vi "main.vi"() -> ()   [LabVIEW 2020]
uses:
  Var/Queue elements.ctl
  Var/Queue elements 2.ctl
  Var/Global 1.vi
  user32.dll
panel:
  out "Примерное время \nобработки":string
  out "2_stan":refnum<queue>
  out "Flag":bool
  out "Curs":refnum<queue>
  out "Progress":i32(slide) scale=-1.0..500.0
  in  "Количество брака":i32 caption="Numeric"
  in  "Общее кол-во обработок":i32 caption="Numeric"
  in  "Close":bool
  out "ERROR":string
  out "Boolean":bool
  in  "Start":bool
  in  "Stop":bool
  in  "error in (no error)":errorcluster
  out "error out":errorcluster
  in  "Объекты":T1={"Ускоренно/Реально"=TRUE, "Станок 1"={"Время на обработку (с)"=40, "Шанс брака (%)"=4.0}, "Станок 2"={"Время на обработку (с)"=60, "Шанс брака (%)"=8.0}, "Кол-во деталей"=500, "Задержки на перемещение"={"Время загрузки\n первого станка (с)"=5, "Время загрузки\n второго станка (с) "=6, "Время до урны (с)"=3, "Время до коробки (с)"=2, "Время между станками (с)"=3}, "Повторная \nобработка\n на станке:"=TRUE}
  # "1"
  # "2"
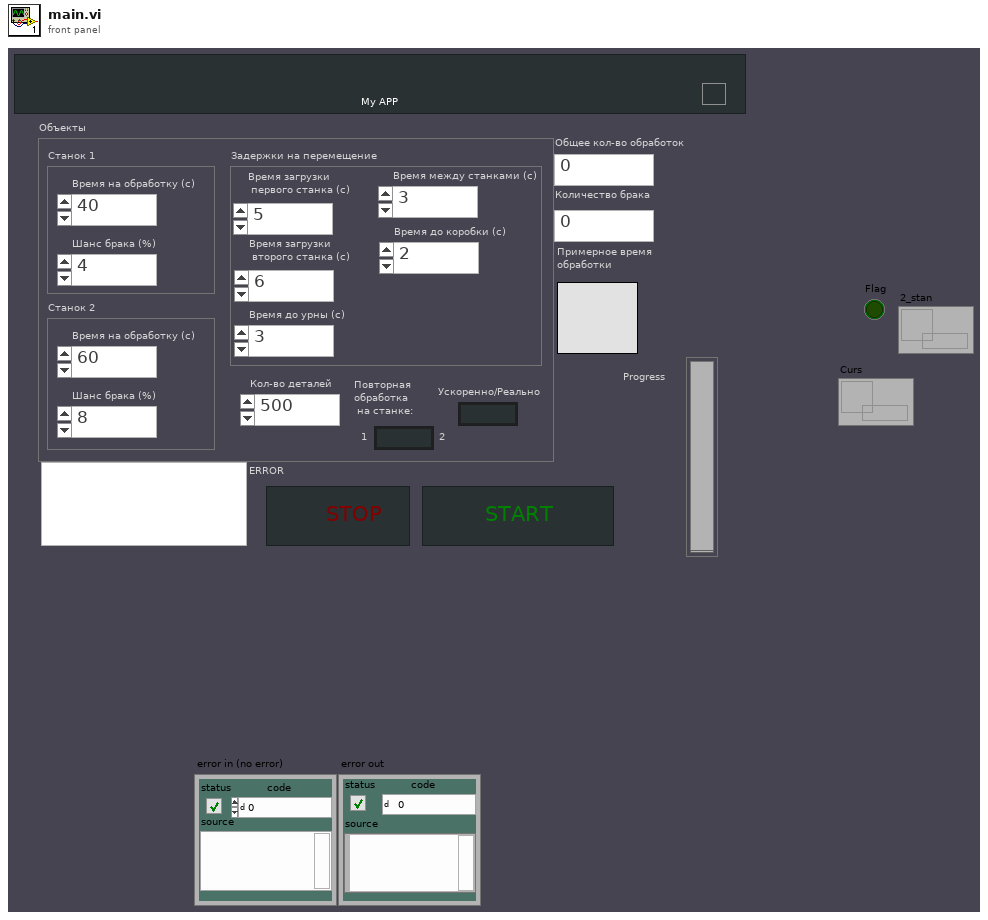
[diagram p1: front panel]
types:
  T1 = cluster{"Ускоренно/Реально":bool, "Станок 1":cluster{"Время на обработку (с)":i32, "Шанс брака (%)":dbl}, "Станок 2":cluster{"Время на обработку (с)":i32, "Шанс брака (%)":dbl}, "Кол-во деталей":i32, "Задержки на перемещение":cluster{"Время загрузки\n первого станка (с)":i32, "Время загрузки\n второго станка (с) ":i32, "Время до урны (с)":i32, "Время до коробки (с)":i32, "Время между станками (с)":i32}, "Повторная \nобработка\n на станке:":bool}
  T2 = typedef "Queue elements 2.ctl" = enum16{"START", "STOP", "CLOSE", "CLEAR"}
  T3 = typedef "Queue elements.ctl" = enum16{"STOP", "START", "CLOSE"}
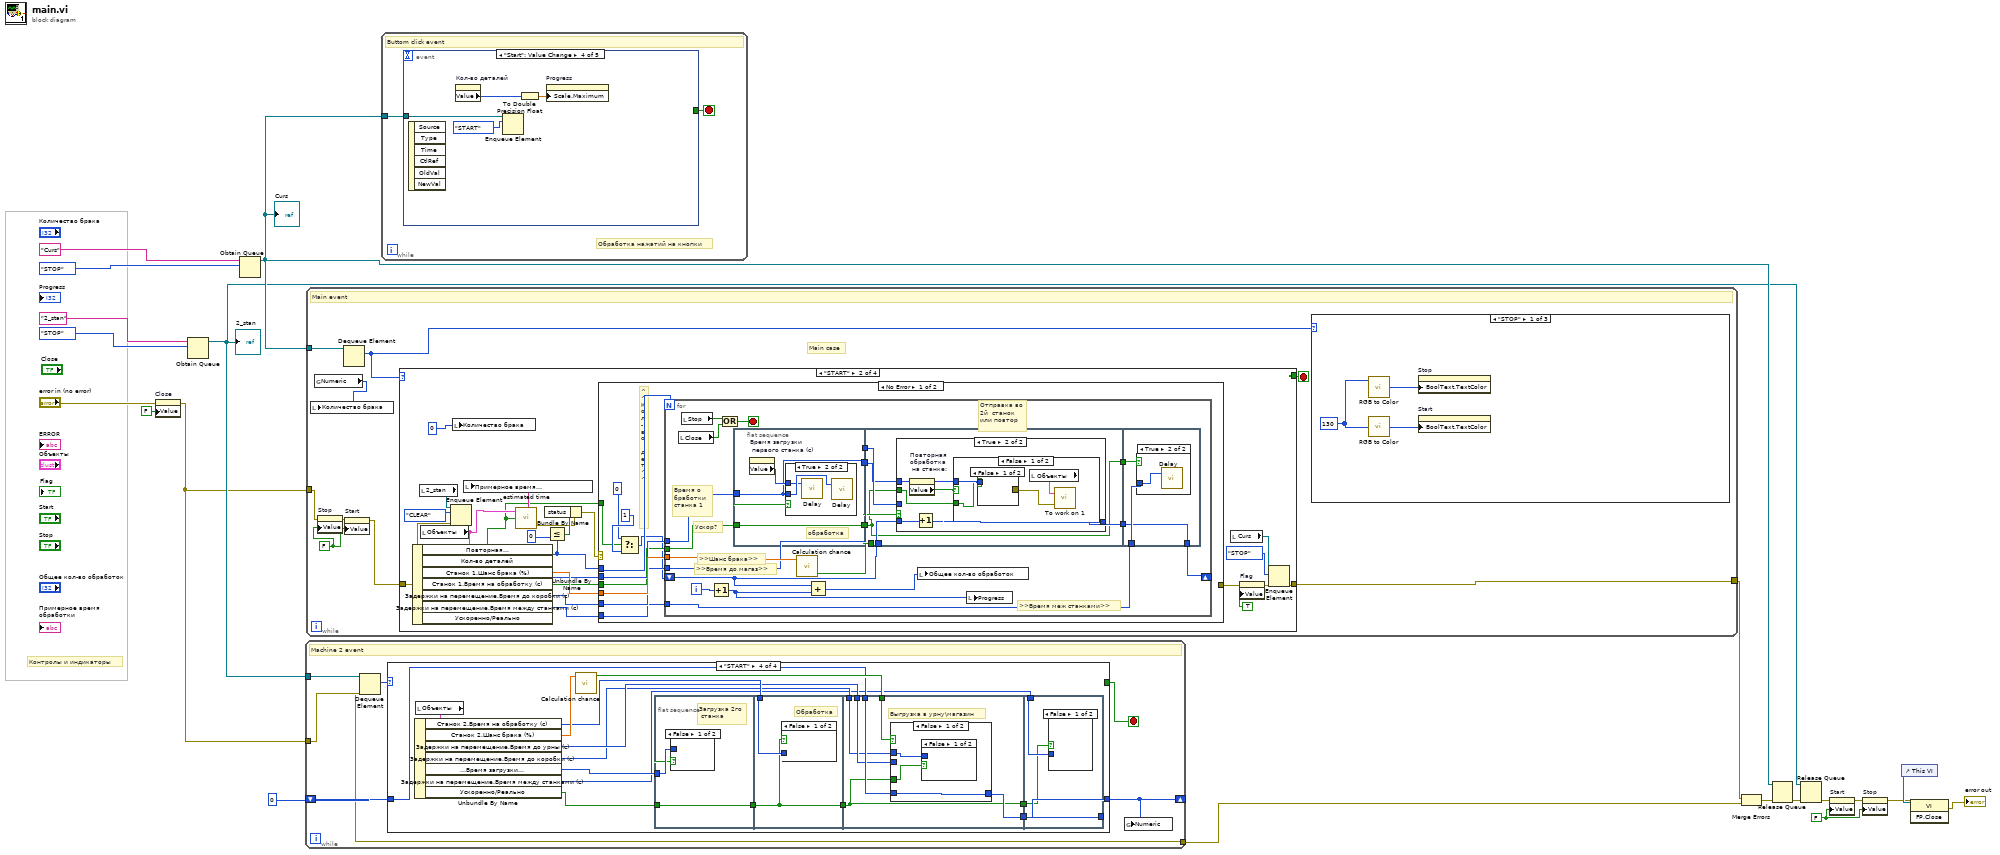
[diagram p0: block diagram]
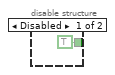
[diagram p3: hidden frame]
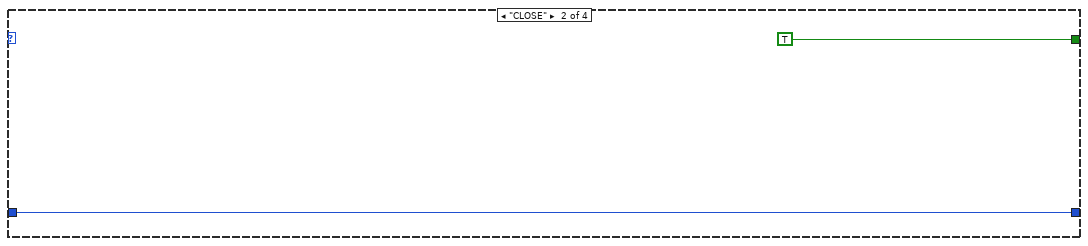
[diagram p4: hidden frame]
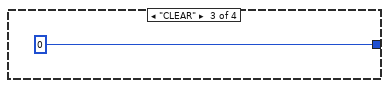
[diagram p5: hidden frame]
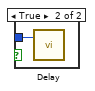
[diagram p6: hidden frame]
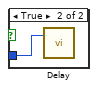
[diagram p7: hidden frame]
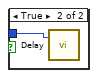
[diagram p8: hidden frame]
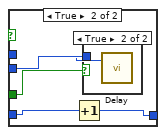
[diagram p9: hidden frame]
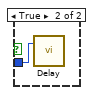
[diagram p11: hidden frame]
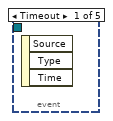
[diagram p12: hidden frame]
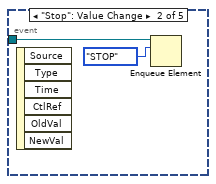
[diagram p13: hidden frame]
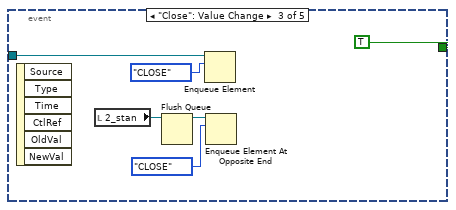
[diagram p14: hidden frame]
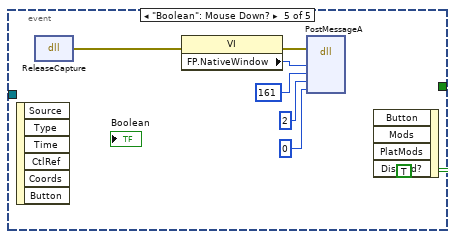
[diagram p15: hidden frame]
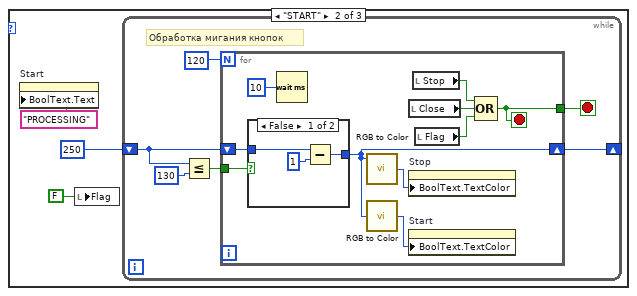
[diagram p16: hidden frame]
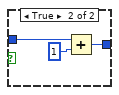
[diagram p17: hidden frame]
diagram:
  w16 = FALSE ("Text Only Button")
  # "Контролы и индикаторы"
  n1 = property on="Close" class="Bool (strict)"(error in="error in (no error)", "Value"=FALSE ("Close")) -> (error out=w5:errorcluster)  [unwired: 1 in, 1 out]
  n2 = Obtain Queue(name (unnamed)="2_stan", element data type=Queue_elements_2."STOP" ("element")) -> (queue out=w9:refnum<queue>)  [unwired: 3 in, 2 out]
  "2_stan" <- w9
  n3 = Obtain Queue(name (unnamed)="Curs", element data type=Queue_elements."STOP") -> (queue out=w18:refnum<queue>)  [unwired: 3 in, 2 out]
  "Curs" <- w18
  n4 = while {
    tunnel: w9 -> [w25]
    shift-right: [w21] -> _
    shift-left: 0 -> [w24]
    tunnel: [w22] -> w6
    tunnel: w5 -> [w23]
    stop <- w26 stop-if-true
    # "Machine 2 event"
    n5 = Dequeue Element(queue=w25, error in (no error)=w23) -> (element=w27:T2, error out=w22:errorcluster)  [unwired: 1 in, 2 out]
    n6 = case shown="\"START\"" w27 {
      tunnel: [w29 TRUE _ _] -> w26
      tunnel: w24 -> [w28 w31 _ w44]
      tunnel: [w28 w31 0 w41] -> w21
      frame "STOP" {
        n7 = disable-structure shown="Enabled" {
          disable-tunnel: [TRUE _] -> w29
          frame Disabled {
          }
          frame Enabled {
          }
        }
      }
      frame "CLOSE" {
      }
      frame "CLEAR" {
      }
      frame "START" {
        n8 = local read "Объекты"() -> (w48:T1)
        n9 = Unbundle By Name(w48) -> ("Станок 2.Время на обработку (с)"=w46:i32, "Станок 2.Шанс брака (%)"=w47:dbl, "Задержки на перемещение.Время до урны (с)"=w43:i32, "Задержки на перемещение.Время до коробки (с)"=w42:i32, "Задержки на перемещение.Время загрузки\n второго станка (с)"=w40:i32, "Задержки на перемещение.Время между станками (с)"=w38:i32, "Ускоренно/Реально"=w34:bool)
        n10 = call "Calculation chance.vi"("Defective (%)"=w47) -> ("Defect"=w45:bool)  [unwired: 1 in]
        n11 = flat-sequence {
          tunnel: w40 -> [w50]
          tunnel: w34 -> [w49]
          tunnel: [w49] -> w37
          tunnel: w46 -> [w53]
          tunnel: w37 -> [w52]
          tunnel: [w52] -> w36
          tunnel: w45 -> [w60]
          tunnel: w44 -> [w59]
          tunnel: w43 -> [w58]
          tunnel: w42 -> [w57]
          tunnel: [w56] -> w39
          tunnel: w36 -> [w55]
          tunnel: [w55] -> w35
          tunnel: [w72] -> w41
          tunnel: w39 -> [w72]
          tunnel: w38 -> [w71]
          tunnel: w35 -> [w70]
          frame #0 {
            # "Загрузка 2го\n станка"
            n12 = case shown="False" w49 {
              tunnel: w50 -> [_ w51]
              frame False {
              }
              frame True {
                n13 = call "Delay.vi"("Wait (s)"=w51) -> ()  [unwired: 1 in, 1 out]
              }
            }
          }
          frame #1 {
            # "Обработка"
            n14 = case shown="False" w52 {
              tunnel: w53 -> [_ w54]
              frame False {
              }
              frame True {
                n15 = call "Delay.vi"("Wait (s)"=w54) -> ()  [unwired: 1 in, 1 out]
              }
            }
          }
          frame #2 {
            # "Выгрузка в урну\\магазин"
            n16 = case shown="False" w60 {
              tunnel: w59 -> [w63 w68]
              tunnel: [w63 w67] -> w56
              tunnel: w58 -> [_ w66]
              tunnel: w57 -> [w62 _]
              tunnel: w55 -> [w61 w65]
              frame False {
                n17 = case shown="False" w61 {
                  tunnel: w62 -> [_ w64]
                  frame False {
                  }
                  frame True {
                    n18 = call "Delay.vi"("Wait (s)"=w64) -> ()  [unwired: 1 in, 1 out]
                  }
                }
              }
              frame True {
                n19 = Increment(x=w68) -> (x+1=w67:i32)
                n20 = case shown="True" w65 {
                  tunnel: w66 -> [_ w69]
                  frame False {
                  }
                  frame True {
                    n21 = call "Delay.vi"("Wait (s)"=w69) -> ()  [unwired: 1 in, 1 out]
                  }
                }
              }
            }
          }
          frame #3 {
            n22 = case shown="False" w70 {
              tunnel: w71 -> [_ w73]
              frame False {
              }
              frame True {
                n23 = call "Delay.vi"("Wait (s)"=w73) -> ()  [unwired: 1 in, 1 out]
              }
            }
          }
        }
      }
    }
    n24 = global write "Global 1.vi" "Numeric"(w21) -> ()
  }
  n25 = while {
    tunnel: [w81] -> w7
    tunnel: w5 -> [w78]
    tunnel: w18 -> [w82]
    stop <- w80 stop-if-true
    w76 = FALSE ("Stop")
    # "Main case"
    # "Main event"
    n26 = global read "Global 1.vi" "Numeric"() -> (w77:i32)
    n27 = local write "Количество брака"(w77) -> ()
    n28 = property on="Stop" class="Bool (strict)"(error in=w78, "Value"=w76) -> (error out=w75:errorcluster)  [unwired: 1 in, 1 out]
    n29 = Dequeue Element(queue=w82) -> (element=w79:T3)  [unwired: 2 in, 3 out]
    n30 = property on="Start" class="Bool (strict)"(error in=w75, "Value"=w76) -> (error out=w74:errorcluster)  [unwired: 1 in, 1 out]
    n31 = case shown="\"START\"" w79 {
      tunnel: w74 -> [w111 w131 w202 w204]
      tunnel: [w111 w128 w201 w204] -> w81
      tunnel: [_ _ _ TRUE] -> w80
      frame Default {
      }
      frame "START" {
        n32 = local read "2_stan"() -> (w123:refnum<queue>)
        n33 = local read "Объекты"() -> (w117:T1)
        n34 = Unbundle By Name(w117) -> ("Повторная \nобработка\n на станке:"=w113:bool, "Кол-во деталей"=w118:i32, "Станок 1.Шанс брака (%)"=w132:dbl, "Станок 1.Время на обработку (с)"=w119:i32, "Задержки на перемещение.Время до коробки (с)"=w122:i32, "Задержки на перемещение.Время между станками (с)"=w121:i32, "Ускоренно/Реально"=w120:bool)
        n35 = Enqueue Element(queue=w123, element=Queue_elements_2."CLEAR", error in (no error)=w131) -> ()  [unwired: 1 in, 3 out]
        n36 = local write "Количество брака"(0 ("Numeric")) -> ()
        n37 = call "estimated time.vi"("Boolean"=w113, "Объекты 2"=w117) -> ("error out"=w115:errorcluster, "Время"=w116:string)  [unwired: 2 in]
        n38 = local write "Примерное время \nобработки"(w116) -> ()
        n39 = Less Or Equal?(x=w118, y=0) -> (x <= y?=w133:bool)
        n40 = Bundle By Name(cluster=w115, "status"=w133) -> (w114:errorcluster)
        n41 = case shown="No Error" w114 {
          selector: w114 -> [_ w200]
          tunnel: [_ w196] -> w127
          tunnel: w132 -> [w143 _]
          tunnel: w118 -> [w144 _]
          tunnel: w119 -> [w142 _]
          tunnel: w122 -> [w141 _]
          tunnel: w121 -> [w140 _]
          tunnel: w120 -> [w139 _]
          tunnel: w113 -> [w135 _]
          frame No Error {
            # "^\n^\nК\nо\nл\n-\nв\nо\n\nд\nе\nт\n^\n^"
            n42 = Select(t=0, s=w135, f=1) -> (s? t:f=w138:i32)
            n43 = for {
              N: w144 -> [_]
              tunnel: w143 -> [w162]
              tunnel: w142 -> [w161]
              shift-right: [w154] -> _
              shift-left: w138 -> [w155]
              tunnel: w141 -> [w153]
              tunnel: w140 -> [w146]
              tunnel: w139 -> [w149]
              i -> [w151]
              stop <- w159 stop-if-true
              # "Отправка во\n2й  станок\nили повтор"
              # ">>Время меж станками>>"
              # ">>Время до магаз>>"
              # ">>Шанс брака>>"
              # "Ускор?"
              # "Время о\nбработки \nстанка 1"
              n44 = local read "Close"() -> (w157:bool)
              n45 = local read "Stop"() -> (w158:bool)
              n46 = Increment(x=w151) -> (x+1=w150:i32)
              n47 = Or(x=w158, y=w157) -> (x .or. y?=w159:bool)
              n48 = flat-sequence {
                tunnel: w161 -> [w163]
                tunnel: w149 -> [w165]
                tunnel: [w165] -> w148
                tunnel: [w163] -> w145
                tunnel: w156 -> [w173]
                tunnel: w155 -> [w172]
                tunnel: w153 -> [w170]
                tunnel: [w171] -> w152
                tunnel: w148 -> [w169]
                tunnel: [w169] -> w147
                tunnel: w145 -> [w168]
                tunnel: [w191] -> w154
                tunnel: w152 -> [w191]
                tunnel: w147 -> [w193]
                tunnel: w146 -> [w192]
                frame #0 {
                  # "обработка"
                  n49 = property on="Время загрузки\n первого станка (с)" class="DigNum (strict)"() -> ("Value"=w164:i32)  [unwired: 2 in, 2 out]
                  n50 = case shown="True" w165 {
                    tunnel: w163 -> [_ w167]
                    tunnel: w164 -> [_ w166]
                    frame False {
                    }
                    frame True {
                      n51 = call "Delay.vi"("Wait (s)"=w166) -> ()  [unwired: 1 in, 1 out]
                      n52 = call "Delay.vi"("Wait (s)"=w167) -> ()  [unwired: 1 in, 1 out]
                    }
                  }
                }
                frame #1 {
                  n53 = case shown="True" w173 {
                    tunnel: w172 -> [w176 w182]
                    tunnel: [w176 w181] -> w171
                    tunnel: w170 -> [w175 _]
                    tunnel: w169 -> [w174 w178]
                    tunnel: w168 -> [_ w179]
                    frame False {
                      # "Время на \nперемещение \nдо\nмагазина"
                      n54 = case shown="True" w174 {
                        tunnel: w175 -> [_ w177]
                        frame False {
                        }
                        frame True {
                          n55 = call "Delay.vi"("Wait (s)"=w177) -> ()  [unwired: 1 in, 1 out]
                        }
                      }
                    }
                    frame True {
                      n56 = property on="Повторная \nобработка\n на станке:" class="Bool (strict)"() -> ("Value"=w180:bool)  [unwired: 2 in, 2 out]
                      n57 = Increment(x=w182) -> (x+1=w181:i32)
                      n58 = case shown="False" w180 {
                        tunnel: w179 -> [w186 _]
                        tunnel: w178 -> [w183 _]
                        frame False {
                          n59 = case shown="False" w183 {
                            tunnel: w186 -> [_ w188]
                            tunnel: [_ w187] -> w185
                            frame False {
                            }
                            frame True {
                              n60 = call "Delay.vi"("Wait (s)"=w188) -> ("error out"=w187:errorcluster)  [unwired: 1 in]
                            }
                          }
                          n61 = local read "Объекты"() -> (w184:T1)
                          n62 = call "To work on 1.vi"("error in (no error)"=w185, "Объекты"=w184) -> ()  [unwired: 1 out]
                        }
                        frame True {
                          n63 = local read "2_stan"() -> (w189:refnum<queue>)
                          n64 = Enqueue Element(queue=w189, element=Queue_elements_2."START") -> ()  [unwired: 2 in, 3 out]
                        }
                      }
                    }
                  }
                }
                frame #2 {
                  n65 = case shown="True" w193 {
                    tunnel: w192 -> [_ w194]
                    frame False {
                    }
                    frame True {
                      n66 = call "Delay.vi"("Wait (s)"=w194) -> ()  [unwired: 1 in, 1 out]
                    }
                  }
                }
              }
              n67 = call "Calculation chance.vi"("Defective (%)"=w162) -> ("Defect"=w156:bool)  [unwired: 1 in]
              n68 = Add(x=w155, y=w150) -> (x+y=w160:i32)
              n69 = local write "Общее кол-во обработок"(w160) -> ()
              n70 = local write "Progress"(w150) -> ()
            }
          }
          frame Error {
            n71 = Bundle By Name(cluster=w200, "status"=FALSE, "code"=0, "source"="Ошибка, количество аргументов <=0 ") -> (w196:errorcluster)
            n72 = Unbundle By Name(w196) -> ("source"=w195:string)
            n73 = local write "ERROR"(w195) -> ()
          }
        }
        n74 = local read "Curs"() -> (w130:refnum<queue>)
        n75 = property on="Flag" class="Bool (strict)"(error in=w127, "Value"=TRUE ("Flag")) -> (error out=w126:errorcluster)  [unwired: 1 in, 1 out]
        n76 = Enqueue Element(queue=w130, element=Queue_elements."STOP", error in (no error)=w126) -> (error out=w128:errorcluster)  [unwired: 1 in, 2 out]
      }
      frame "STOP" {
        n77 = property on="Start" class="Bool (strict)"(error in=w202, "BoolText.Text"="START" ("Boolean Text.Text")) -> (error out=w201:errorcluster)  [unwired: 1 in, 1 out]
      }
      frame "CLOSE" {
      }
    }
    n78 = case shown="\"STOP\"" w79 {
      frame "STOP" {
        w83 = u8 130 ("G")
        n79 = call <vilib>:"RGB to Color.vi"("R"=w83) -> ("Color"=w85:u32)  [unwired: 2 in]
        n80 = call <vilib>:"RGB to Color.vi"("G"=w83) -> ("Color"=w84:u32)  [unwired: 2 in]
        n81 = property on="Stop" class="Bool (strict)"("BoolText.TextColor"=w85) -> ()  [unwired: 2 in, 2 out]
        n82 = property on="Start" class="Bool (strict)"("BoolText.TextColor"=w84) -> ()  [unwired: 2 in, 2 out]
      }
      frame "START" {
        n83 = property on="Start" class="Bool (strict)"("BoolText.Text"="PROCESSING" ("Boolean Text.Text")) -> ()  [unwired: 2 in, 2 out]
        n84 = local write "Flag"(FALSE ("Flag")) -> ()
        n85 = while {
          shift-right: [w92] -> _
          shift-left: u8 250 ("R") -> [w93]
          stop <- w89 stop-if-true
          # "Обработка мигания кнопок"
          n86 = Less Or Equal?(x=w93, y=u8 130) -> (x <= y?=w90:bool)
          n87 = for {
            N: 120 -> [_]
            shift-right: [w99] -> w92
            shift-left: w93 -> [w103]
            tunnel: w90 -> [w102]
            tunnel: [w96] -> w89
            stop <- w96 stop-if-true
            n88 = case shown="False" w102 {
              tunnel: [w107 w110] -> w99
              tunnel: w103 -> [w106 w109]
              frame False {
                n89 = Subtract(x=w106, y=u8 1) -> (x-y=w107:u8)
              }
              frame True {
                n90 = Add(x=w109, y=u8 1) -> (x+y=w110:u8)
              }
            }
            n91 = Wait (ms)(milliseconds to wait=u32 10) -> ()  [unwired: 1 out]
            n92 = call <vilib>:"RGB to Color.vi"("R"=w99) -> ("Color"=w104:u32)  [unwired: 2 in]
            n93 = call <vilib>:"RGB to Color.vi"("G"=w99) -> ("Color"=w100:u32)  [unwired: 2 in]
            n94 = local read "Close"() -> (w97:bool)
            n95 = property on="Stop" class="Bool (strict)"("BoolText.TextColor"=w104) -> ()  [unwired: 2 in, 2 out]
            n96 = property on="Start" class="Bool (strict)"("BoolText.TextColor"=w100) -> ()  [unwired: 2 in, 2 out]
            n97 = local read "Stop"() -> (w98:bool)
            n98 = local read "Flag"() -> (w95:bool)
            n99 = Compound Arithmetic op=OR(w98, w97, w95) -> (w96:bool)
          }
        }
      }
      frame "CLOSE" {
      }
    }
  }
  n100 = while {
    tunnel: w18 -> [w206]
    stop <- w207 stop-if-true
    # "Обработка нажатий на кнопки"
    # "Buttom click event"
    n101 = event shown="[3] \"Start\": Value Change" {
      selector: _ -> [_ _ _ _ _]
      dyn-events: _ -> [_ _ _ _ _]
      timeout: _ -> [_ _ _ _ _]
      tunnel: w206 -> [_ w208 w213 w218 _]
      tunnel: [_ _ TRUE _ _] -> w207
      event Timeout {
        n102 = event-data() -> ()  [unwired: 1 in, 3 out]
      }
      event "Stop": Value Change {
        n103 = event-data() -> ()  [unwired: 1 in, 6 out]
        n104 = Enqueue Element(queue=w208, element=Queue_elements."STOP") -> ()  [unwired: 2 in, 3 out]
      }
      event "Close": Value Change {
        n105 = event-data() -> ()  [unwired: 1 in, 6 out]
        n106 = local read "2_stan"() -> (w211:refnum<queue>)
        n107 = Flush Queue(queue=w211) -> (queue out=w210:refnum<queue>)  [unwired: 1 in, 2 out]
        n108 = Enqueue Element(queue=w213, element=Queue_elements."CLOSE") -> ()  [unwired: 2 in, 3 out]
        n109 = Enqueue Element At Opposite End(queue=w210, element=Queue_elements_2."CLOSE") -> ()  [unwired: 2 in, 3 out]
      }
      event "Start": Value Change {
        n110 = event-data() -> ()  [unwired: 1 in, 6 out]
        n111 = property on="Кол-во деталей" class="DigNum (strict)"() -> ("Value"=w216:i32)  [unwired: 2 in, 2 out]
        n112 = Enqueue Element(queue=w218, element=Queue_elements."START") -> ()  [unwired: 2 in, 3 out]
        n113 = To Double Precision Float(number=w216) -> (double precision float=w217:dbl)
        n114 = property on="Progress" class="Slide (strict)"("Scale.Maximum"=w217) -> ()  [unwired: 2 in, 2 out]
      }
      event "Boolean": Mouse Down? {
        n115 = event-data() -> ()  [unwired: 1 in, 6 out]
        n116 = dll-call lib="user32.dll" fn="ReleaseCapture"() -> (error out=w225:errorcluster)  [unwired: 4 in, 1 out]
        n117 = property class="VI"(error in=w225) -> (error out=w224:errorcluster, "FP.NativeWindow"=w223:u64)  [unwired: 1 in, 1 out]
        n118 = dll-call lib="user32.dll" fn="PostMessageA"(error in=w224, "hWnd"=w223, "Msg"=161, "wParam"=2, "lParam"=0) -> ()  [unwired: 7 in, 2 out]
        n119 = event-data("Discard?"=TRUE) -> ()  [unwired: 4 in, 1 out]
      }
    }
  }
  n120 = Merge Errors(w7, w6) -> (w4:errorcluster)
  n121 = Release Queue(queue=w18, error in (no error)=w4) -> (error out=w12:errorcluster)  [unwired: 1 in, 2 out]
  n122 = Release Queue(queue=w9, error in (no error)=w12) -> (error out=w11:errorcluster)  [unwired: 1 in, 2 out]
  n123 = property on="Start" class="Bool (strict)"(error in=w11, "Value"=w16) -> (error out=w17:errorcluster)  [unwired: 1 in, 1 out]
  n124 = property on="Stop" class="Bool (strict)"(error in=w17, "Value"=w16) -> (error out=w2:errorcluster)  [unwired: 1 in, 1 out]
  n125 = control-ref of="This VI"() -> (w3:refnum<vi>)
  n126 = invoke class="VI" method="FP.Close"(reference=w3, error in=w2) -> (error out=→"error out":errorcluster)  [unwired: 1 in, 2 out]
